vi "Pndt 1-4 byte combiner.vi"(1 "#bytes":i32, 2 "start index [0]":i32, 3 "[U8] count bytes":u8[](array[numeric]) format="%.0x") -> (0 "U32":u32 format="%.0x")   [LabVIEW 2026, in "MicroPulse_Driver.lvlib"]
uses:
  MicroPulse_Driver.lvlib
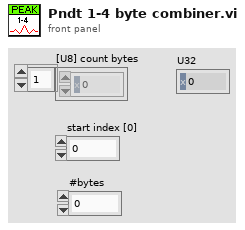
[diagram p1: front panel]
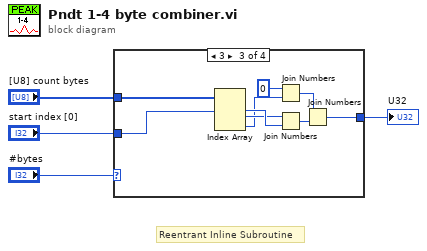
[diagram p0: block diagram]
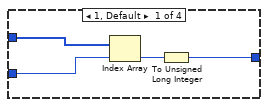
[diagram p2: hidden frame]
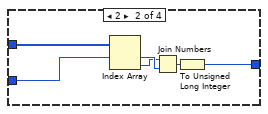
[diagram p3: hidden frame]
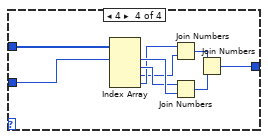
[diagram p4: hidden frame]
diagram:
  # "Reentrant Inline Subroutine"
  n1 = case shown="3" "#bytes" {
    tunnel: [w6 w10 w19 w29] -> w3
    tunnel: "[U8] count bytes" -> [w8 w13 w21 w30]
    tunnel: "start index [0]" -> [w5 w9 w18 w24]
    frame 1, Default {
      n2 = Index Array(array=w8, index=w5) -> (element=w7:u8)
      n3 = To Unsigned Long Integer(number=w7) -> (unsigned 32bit integer=w6:u32)
    }
    frame 2 {
      n4 = Index Array(array=w13, index #1=w9) -> (element #1=w12:u8, element #2=w11:u8)  [unwired: 1 in]
      n5 = Join Numbers(hi=w11, lo=w12) -> ((hi.lo)=w14:u16)
      n6 = To Unsigned Long Integer(number=w14) -> (unsigned 32bit integer=w10:u32)
    }
    frame 3 {
      n7 = Index Array(array=w21, index #1=w18) -> (element #1=w17:u8, element #2=w16:u8, element #3=w15:u8)  [unwired: 2 in]
      n8 = Join Numbers(hi=u8 0, lo=w15) -> ((hi.lo)=w22:u16)
      n9 = Join Numbers(hi=w16, lo=w17) -> ((hi.lo)=w23:u16)
      n10 = Join Numbers(hi=w22, lo=w23) -> ((hi.lo)=w19:u32)
    }
    frame 4 {
      n11 = Index Array(array=w30, index #1=w24) -> (element #1=w28:u8, element #2=w27:u8, element #3=w25:u8, element #4=w26:u8)  [unwired: 3 in]
      n12 = Join Numbers(hi=w26, lo=w25) -> ((hi.lo)=w31:u16)
      n13 = Join Numbers(hi=w27, lo=w28) -> ((hi.lo)=w32:u16)
      n14 = Join Numbers(hi=w31, lo=w32) -> ((hi.lo)=w29:u32)
    }
  }
  "U32" <- w3
